vi "Get Create Test Channel Sensor Names.vi"(8 "error in (no error)":errorcluster, 11 "Abstract Create Test Channel Sensor Names Msg in":refnum<class "Abstract Create Test Channel Sensor Names Msg.lvclass">) -> (0 "error out":errorcluster, 2 "Create Test Channel Sensor Names":string[](array[string]), 3 "Abstract Create Test Channel Sensor Names Msg out":refnum<class "Abstract Create Test Channel Sensor Names Msg.lvclass">)   [LabVIEW 2013, in "Create Test Channel Model.lvlib" / "Abstract Create Test Channel Sensor Names Msg.lvclass"]
uses:
  Abstract Create Test Channel Sensor Names Msg.lvclass
  Abstract Create Test Channel Sensor Names Msg.lvclass/Abstract Create Test Channel Sensor Names Msg.ctl
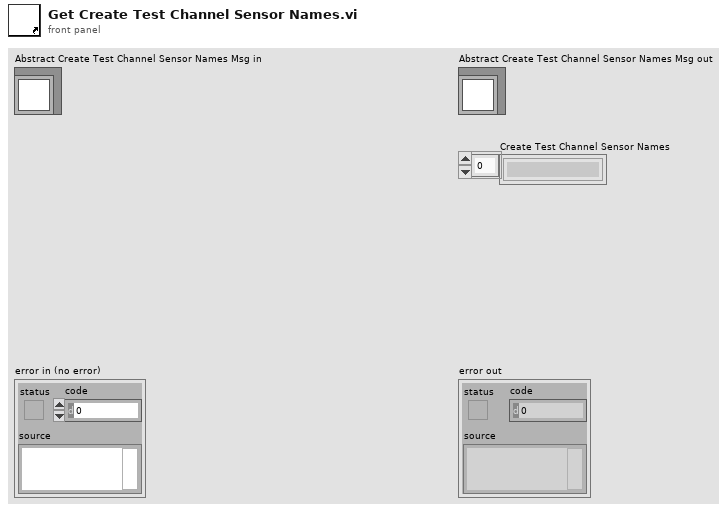
[diagram p1: front panel]
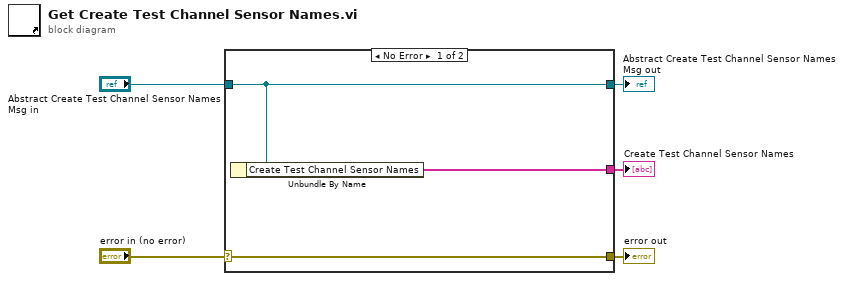
[diagram p0: block diagram]
diagram:
  n1 = case shown="No Error" "error in (no error)" {
    selector: "error in (no error)" -> [w8 w9]
    tunnel: [w8 w9] -> w4
    tunnel: [w7 w10] -> w2
    tunnel: "Abstract Create Test Channel Sensor Names Msg in" -> [w7 w10]
    tunnel: [w6 _] -> w1
    frame No Error {
      n2 = Unbundle By Name(w7) -> ("Create Test Channel Sensor Names"=w6:string[])
    }
    frame Error {
    }
  }
  "error out" <- w4
  "Abstract Create Test Channel Sensor Names Msg out" <- w2
  "Create Test Channel Sensor Names" <- w1
